vi "Exercise 7.1_Normal_Answer.vi"() -> ()   [LabVIEW 2010]
uses:
  7.1 States.ctl
panel:
  in  "Stop":bool
  out "Walk Sign":bool
  out "Green":bool
  out "Yellow":bool
  out "Red":bool
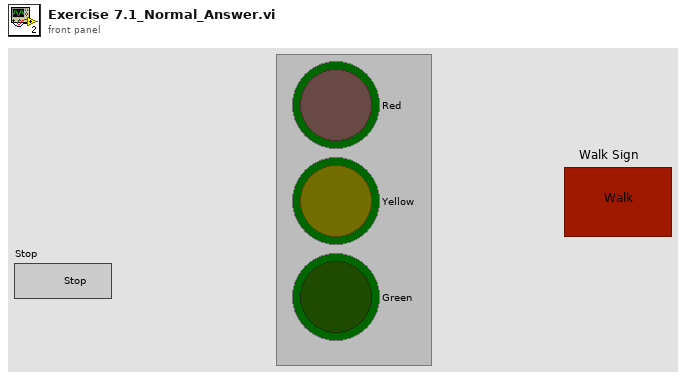
[diagram p1: front panel]
types:
  T1 = typedef "7.1 States.ctl" = enum16{"Initialize", "Green", "Yellow", "Red 1", "Red 2", "Stop"}
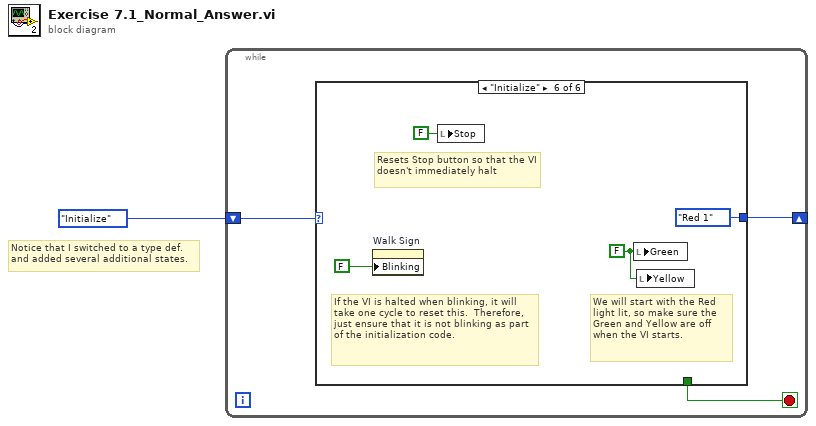
[diagram p0: block diagram]
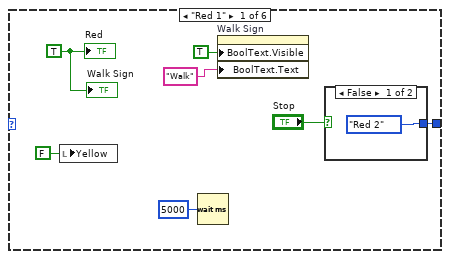
[diagram p2: hidden frame]
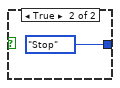
[diagram p3: hidden frame]
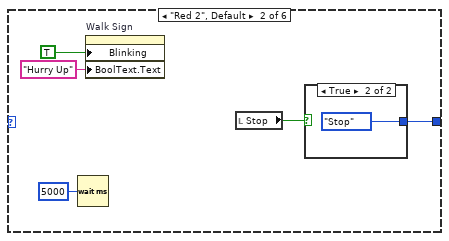
[diagram p4: hidden frame]
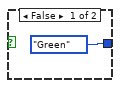
[diagram p5: hidden frame]
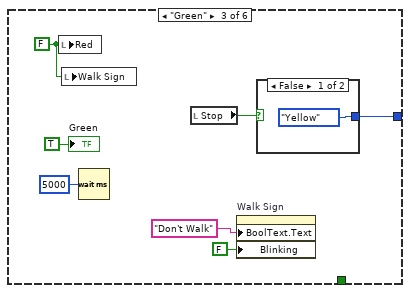
[diagram p6: hidden frame]
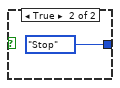
[diagram p7: hidden frame]
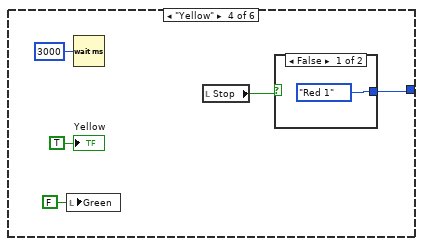
[diagram p8: hidden frame]
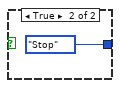
[diagram p9: hidden frame]
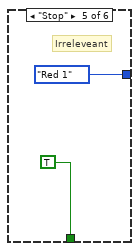
[diagram p10: hidden frame]
diagram:
  # "Notice that I switched to a type def.\nand added several additional states."
  n1 = while {
    shift-right: [w3] -> _
    shift-left: 7.1_States."Initialize" -> [w4]
    stop <- w2 stop-if-true
    n2 = case shown="\"Initialize\"" w4 {
      tunnel: [w7 w16 w23 w32 7.1_States."Red 1" 7.1_States."Red 1"] -> w3
      tunnel: [_ _ _ _ TRUE _] -> w2
      frame "Red 1" {
        w10 = TRUE ("Red")
        n3 = local write "Yellow"(FALSE ("Yellow")) -> ()
        n4 = Wait (ms)(milliseconds to wait=u32 5000) -> ()  [unwired: 1 out]
        n5 = property on="Walk Sign" class="Bool"("BoolText.Visible"=TRUE ("Boolean Text.Visible"), "BoolText.Text"="Walk" ("Boolean Text.Text")) -> ()  [unwired: 2 in, 2 out]
        n6 = case shown="False" "Stop" {
          tunnel: [7.1_States."Red 2" 7.1_States."Stop"] -> w7
          frame False {
          }
          frame True {
          }
        }
        "Red" <- w10
        "Walk Sign" <- w10
      }
      frame "Red 2", Default {
        n7 = Wait (ms)(milliseconds to wait=u32 5000) -> ()  [unwired: 1 out]
        n8 = property on="Walk Sign" class="Bool"("Blinking"=TRUE, "BoolText.Text"="Hurry Up" ("Boolean Text.Text")) -> ()  [unwired: 2 in, 2 out]
        n9 = local read "Stop"() -> (w15:bool)
        n10 = case shown="True" w15 {
          tunnel: [7.1_States."Green" 7.1_States."Stop"] -> w16
          frame False {
          }
          frame True {
          }
        }
      }
      frame "Green" {
        w27 = FALSE ("Red")
        n11 = local write "Red"(w27) -> ()
        n12 = local write "Walk Sign"(w27) -> ()
        n13 = Wait (ms)(milliseconds to wait=u32 5000) -> ()  [unwired: 1 out]
        n14 = local read "Stop"() -> (w22:bool)
        n15 = property on="Walk Sign" class="Bool"("BoolText.Text"="Don't Walk" ("Boolean Text.Text"), "Blinking"=FALSE) -> ()  [unwired: 2 in, 2 out]
        n16 = case shown="False" w22 {
          tunnel: [7.1_States."Yellow" 7.1_States."Stop"] -> w23
          frame False {
          }
          frame True {
          }
        }
        "Green" <- TRUE ("Green")
      }
      frame "Yellow" {
        n17 = local write "Green"(FALSE ("Green")) -> ()
        n18 = Wait (ms)(milliseconds to wait=u32 3000) -> ()  [unwired: 1 out]
        n19 = local read "Stop"() -> (w31:bool)
        n20 = case shown="False" w31 {
          tunnel: [7.1_States."Red 1" 7.1_States."Stop"] -> w32
          frame False {
          }
          frame True {
          }
        }
        "Yellow" <- TRUE ("Yellow")
      }
      frame "Stop" {
        # "Irreleveant"
      }
      frame "Initialize" {
        w39 = FALSE ("Green")
        # "We will start with the Red light lit, so make sure the Green and Yellow are off when the VI starts."
        # "If the VI is halted when blinking, it will take one cycle to reset this.  Therefore, just ensure that it is not blinking as part of the initialization code."
        # "Resets Stop button so that the VI doesn't immediately halt"
        n21 = property on="Walk Sign" class="Bool"("Blinking"=FALSE) -> ()  [unwired: 2 in, 2 out]
        n22 = local write "Stop"(FALSE ("Stop")) -> ()
        n23 = local write "Green"(w39) -> ()
        n24 = local write "Yellow"(w39) -> ()
      }
    }
  }
